vi "AmbientTemp.vi"(1 "Biome Temperature":dbl) -> (15 "Biome Ambient Temp (K)":dbl)   [LabVIEW 2023]
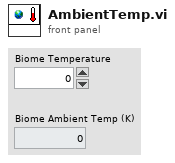
[diagram p1: front panel]
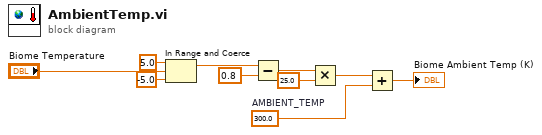
[diagram p0: block diagram]
diagram:
  w3 = 300.0  # AMBIENT_TEMP
  n1 = In Range and Coerce(upper limit=5.0, x="Biome Temperature", lower limit=-5.0) -> (coerced(x)=w7:dbl)  [unwired: 1 out]
  n2 = Subtract(x=w7, y=0.8) -> (x-y=w5:dbl)
  n3 = Multiply(x=w5, y=25.0) -> (x*y=w2:dbl)
  n4 = Add(x=w2, y=w3) -> (x+y=→"Biome Ambient Temp (K)":dbl)
